vi "Example cRIO Master FPGA.vi"() -> ()   [LabVIEW 2012]
uses:
  <vilib>/rvi/eio/common/nirviEmuTemplateMethod_errors.vi
  <vilib>/eio/EIONode/EIONode.xnode
panel:
  out "Heartbeat":bool
  in  "Enable\nDrive":bool
  out "Encoder Position":i32
  in  "stop":bool
  in  "Count(mSec)":u32
  out "Setpoint (Deg)":fxp<+/-,33,11>
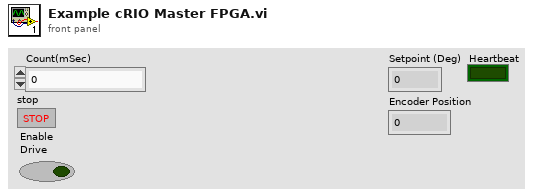
[diagram p1: front panel]
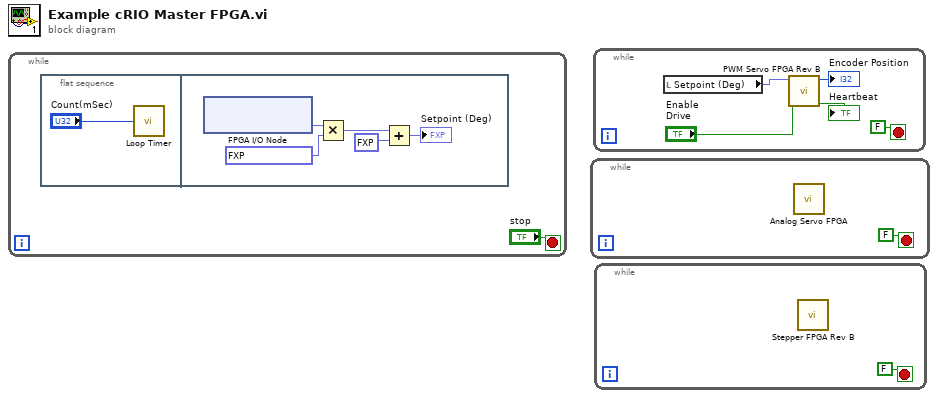
[diagram p0: block diagram]
diagram:
  n1 = while {
    stop <- "stop" stop-if-true
    n2 = flat-sequence {
      frame #0 {
        n3 = call "Loop Timer"("Count(mSec)"="Count(mSec)") -> ()  [unwired: 1 out]
      }
      frame #1 {
        n4 = xnode "FPGA I/O Node"() -> ("Setpoint Pot"=w7:fxp<+/-,16,5>)  [unwired: 1 in, 1 out]
        n5 = Multiply(x=w7, y=fxp<+/-,16,5> 15.99951171875) -> (x*y=w6:fxp<+/-,32,10>)
        n6 = Add(x=w6, y=fxp<+/-,32,10> 123.0) -> (x+y=→"Setpoint (Deg)":fxp<+/-,33,11>)
      }
    }
  }
  n7 = while {
    stop <- FALSE stop-if-true
    n8 = call "Analog Servo FPGA.vi"() -> ()  [unwired: 10 in, 2 out]
  }
  n9 = while {
    stop <- FALSE stop-if-true
    n10 = local read "Setpoint (Deg)"() -> (w12:fxp<+/-,33,11>)
    n11 = call "PWM Servo FPGA Rev B.vi"("Enable\nDrive"="Enable\nDrive", "Position Setpoint"=w12) -> ("Trig AI"=→"Heartbeat":bool, "Encoder Position"=→"Encoder Position":i32)  [unwired: 7 in]
  }
  n12 = while {
    stop <- FALSE stop-if-true
    n13 = call "Stepper FPGA Rev B.vi"() -> ()  [unwired: 12 in]
  }
